vi "_Dummy.vi"   [LabVIEW 2023, in "QHull.lvlib"]
uses:
  QHull.lvlib
  qhull_r_64.dll
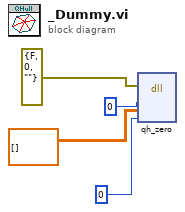
[diagram p0: block diagram]
diagram:
  n1 = dll-call lib="E:/Labview/LV 2023/PPL/PPL Builder/Libs/SK Spatial/QHull/LV QHull/qhull_r_*.dll" fn="qh_zero"(error in=errorcluster {"status"=FALSE, "code"=0, "source"=""} ("error in (no error)"), "ps"=i64 0, "pd"=dbl[][] [], "size"=i64 0) -> ()  [unwired: 6 in, 2 out]
